vi "split.vi"(10 "strInput":string) -> (0 "length":i32, 1 "datoB":string, 2 "datoA":string, 3 "number":u16[](array[numeric]) format="%.0x", 4 "number2":u16[](array[numeric]) format="%.0x")   [LabVIEW 2017]
panel:
  out "Array":string[](array[string])
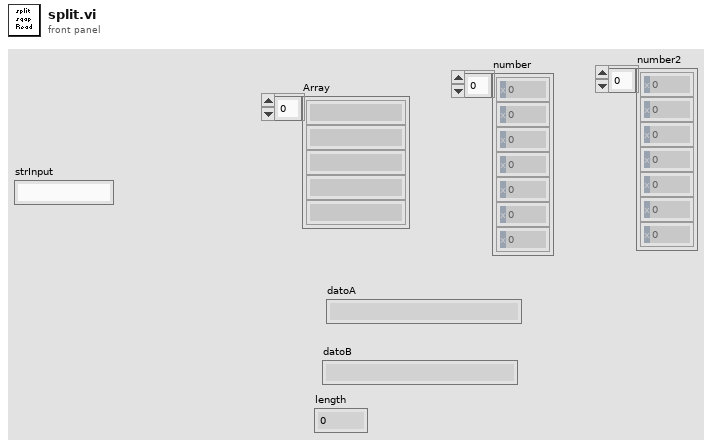
[diagram p1: front panel]
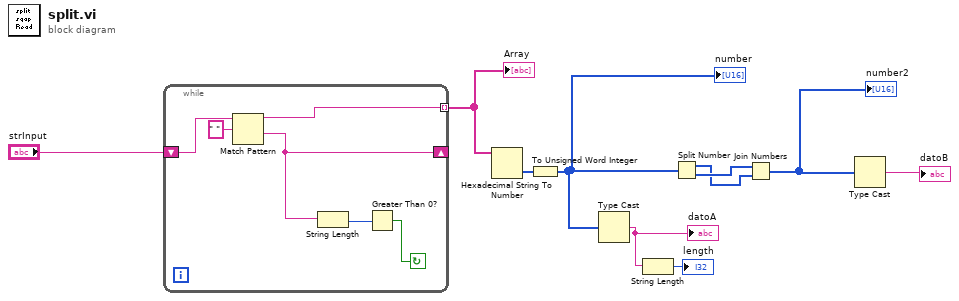
[diagram p0: block diagram]
diagram:
  n1 = while {
    shift-right: [w13] -> _
    shift-left: "strInput" -> [w16]
    tunnel: [w14] -> w9 mode=indexing
    stop <- w11 continue-if-true
    n2 = Match Pattern(string=w16, regular expression=" ") -> (before substring=w14:string, after substring=w13:string)  [unwired: 1 in, 2 out]
    n3 = String Length(string=w13) -> (length=w12:i32)
    n4 = Greater Than 0?(x=w12) -> (x > 0?=w11:bool)
  }
  "Array" <- w9
  n5 = Hexadecimal String To Number(string=w9) -> (number=w8:u32[])  [unwired: 2 in, 1 out]
  n6 = To Unsigned Word Integer(number=w8) -> (unsigned 16bit integer=w5:u16[])
  "number" <- w5
  n7 = Type Cast(x=w5) -> (*(type *) &x=w7:string)  [unwired: 1 in]
  "datoA" <- w7
  n8 = String Length(string=w7) -> (length=→"length":i32)
  n9 = Split Number(x=w5) -> (hi(x)=w3:u8[], lo(x)=w4:u8[])
  n10 = Join Numbers(hi=w4, lo=w3) -> ((hi.lo)=w2:u16[])
  "number2" <- w2
  n11 = Type Cast(x=w2) -> (*(type *) &x=→"datoB":string)  [unwired: 1 in]
